vi "Test 1.vi"() -> ()   [LabVIEW 2016, in "Drona basic.lvlib"]
uses:
  Drona basic.lvlib
  <vilib>/event_ctls.llb/eventsource.ctl
  <vilib>/event_ctls.llb/lveventtype.ctl
  <vilib>/Utility/miscctls.llb/LVPoint32TypeDef.ctl
  <vilib>/Utility/miscctls.llb/LVPositionTypeDef.ctl
  <vilib>/Utility/miscctls.llb/LVBoundsTypeDef.ctl
panel:
  out "Position 2":T1
  out "Bounds 2":T2
  out "Bounds":T2
  out "Position":T1
  out "PlatMods":T3
  out "Mods":cluster{"Double Click":bool, "Menu Key":bool}
  out "Button":u16
  out "Coords":T4
  out "CtlRef":refnum<vi>
  out "Time":u32
  out "Type":T5=enum."Value Change"
  out "Source":T6 items=["LabVIEW UI"=0, "ActiveX"=1, "User Event"=25]
  in  "Cluster":T7 {"Slide" scale=0.0..10.0}
  in  "String":string
  in  "Boolean":bool
  in  "Slide":dbl(slide) scale=0.0..10.0
  in  "Numeric":dbl
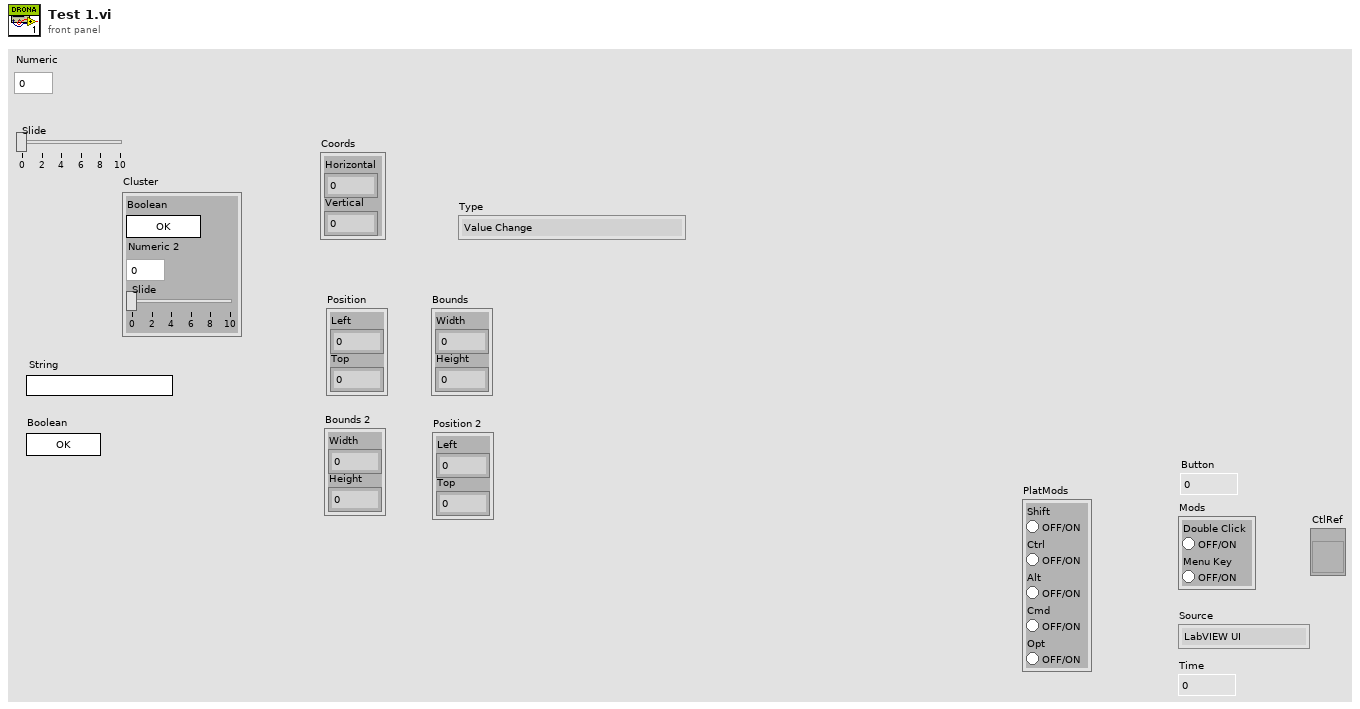
[diagram p1: front panel]
types:
  T1 = typedef "LVPositionTypeDef.ctl" = cluster{"Left":i32, "Top":i32}
  T2 = typedef "LVBoundsTypeDef.ctl" = cluster{"Width":u32, "Height":u32}
  T3 = cluster{"Shift":bool, "Ctrl":bool, "Alt":bool, "Cmd":bool, "Opt":bool}
  T4 = typedef "LVPoint32TypeDef.ctl" = cluster{"Horizontal":i32, "Vertical":i32}
  T5 = typedef "lveventtype.ctl" = enum32{"Null", "Timeout", "Annotation Menu Selection", "Annotation Menu Selection?", "App Instance Close", "App Instance Close?", "Autoscale Range Change", "Bookmark Info Change", "Cell Edit", "Cell Edit?", "Cursor Grab", "Cursor Grab?", "Cursor Menu Selection", "Cursor Menu Selection?", "Cursor Move", "Cursor Release", "Data Change", "Direction Change", "Display State Change", "Drag Ended", "Drag Enter", "Drag Leave", "Drag Over", "Drag Source Update", "Drag Starting", "Drag Starting?", "Drop", "Exec State Change", "Key Down", "Key Down?", "Key Repeat", "Key Repeat?", "Key Up", "Listbox Double Click", "Menu Activation?", "Menu Selection (App)", "Menu Selection? (App)", "Menu Selection (User)", "Mouse Down", "Mouse Down?", "Mouse Enter", "Mouse Leave", "Mouse Move", "Mouse Up", "Mouse Wheel", "NI Security User Change (App)", "Pane Size", "Panel Close", "Panel Close?", "Panel Resize", "Plot Attribute Change", "Scale Range Change", "Shortcut Menu Activation?", "Shortcut Menu Selection (App)", "Shortcut Menu Selection? (App)", "Shortcut Menu Selection (User)", "Tree Double Click", "Tree Drag", "Tree Drag?", "Tree Drop", "Tree Drop?", "Tree Item Close", "Tree Item Close?", "Tree Item Open", "Tree Item Open?", "User Event", "Value Change"}
  T6 = typedef "eventsource.ctl" = u32
  T7 = cluster{"Boolean":bool, "Numeric 2":dbl, "Slide":dbl}
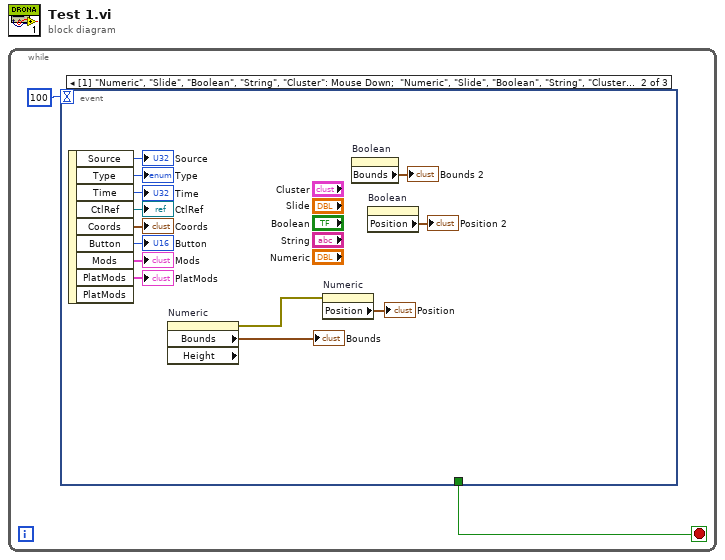
[diagram p0: block diagram]
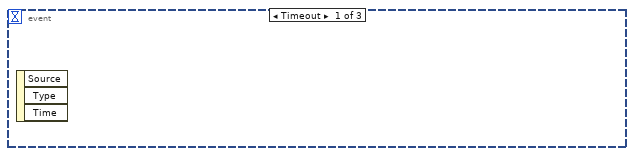
[diagram p2: hidden frame]
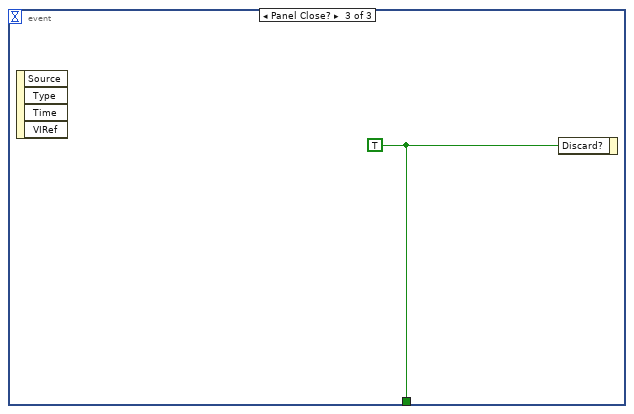
[diagram p3: hidden frame]
diagram:
  n1 = while {
    stop <- w2 stop-if-true
    n2 = event shown="[1] \"Numeric\", \"Slide\", \"Boolean\", \"String\", \"Cluster\": Mouse Down;  \"Numeric\", \"Slide\", \"Boolean\", \"String\", \"Cluster\": Mouse Up" {
      selector: _ -> [_ _ _]
      dyn-events: _ -> [_ _ _]
      timeout: 100 -> [_ _ _]
      tunnel: [_ _ w16] -> w2
      event Timeout {
        n3 = event-data() -> ()  [unwired: 1 in, 3 out]
      }
      event "Numeric", "Slide", "Boolean", "String", "Cluster": Mouse Down; "Numeric", "Slide", "Boolean", "String", "Cluster": Mouse Up {
        n4 = event-data() -> ("Source"=→"Source":T6, "Type"=→"Type":T5, "Time"=→"Time":u32, "CtlRef"=→"CtlRef":refnum<vi>, "Coords"=→"Coords":T4, "Button"=→"Button":u16, "Mods"=→"Mods":cluster{"Double Click":bool, "Menu Key":bool}, "PlatMods"=→"PlatMods":T3)  [unwired: 1 in, 1 out]
        n5 = property on="Numeric" class="DigNum (strict)" props=["Bounds", "Height"]() -> (error out=w7:errorcluster, "Bounds"=→"Bounds":T2)  [unwired: 2 in, 2 out]
        n6 = property on="Numeric" class="DigNum (strict)"(error in=w7) -> ("Position"=→"Position":T1)  [unwired: 1 in, 2 out]
        n7 = property on="Boolean" class="Bool"() -> ("Bounds"=→"Bounds 2":T2)  [unwired: 2 in, 2 out]
        n8 = property on="Boolean" class="Bool"() -> ("Position"=→"Position 2":T1)  [unwired: 2 in, 2 out]
      }
      event Panel Close? {
        w16 = TRUE ("Discard?")
        n9 = event-data() -> ()  [unwired: 1 in, 4 out]
        n10 = event-data("Discard?"=w16) -> ()  [unwired: 1 in, 1 out]
      }
    }
  }
